vi "Self-Calibrate.vi"(8 "error in (no error)":errorcluster, 10 "Timeout (180000)":u32=180000, 11 "VISA resource name":refnum<visa-resource-name>) -> (0 "error out":errorcluster, 2 "Calibration Result":i32, 3 "VISA resource name out":refnum<visa-resource-name>)   [LabVIEW 2015, in "Tektronix TDS 200 1000 2000 Series.lvlib"]
doc: "Calibrates the oscilliscope for acquisitions and measurements."
uses:
  <instrlib>/Tektronix TDS 200 1000 2000 Series/Tektronix TDS 200 1000 2000 Series.lvlib
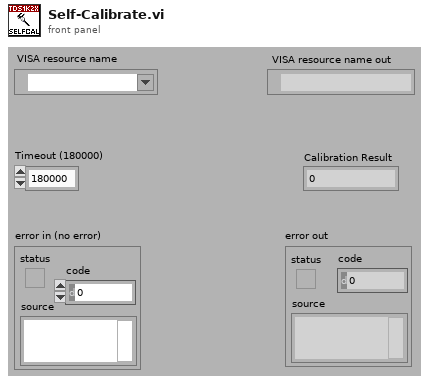
[diagram p1: front panel]
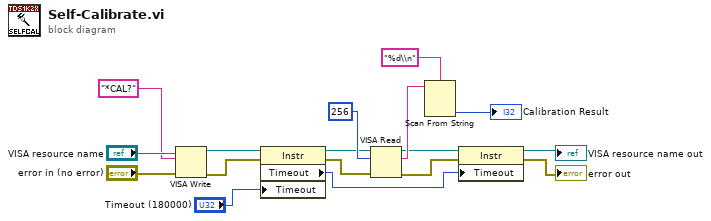
[diagram p0: block diagram]
diagram:
  n1 = VISA Write(VISA resource name="VISA resource name", write buffer="*CAL?", error in (no error)="error in (no error)") -> (VISA resource name out=w10:refnum<visa-resource-name>, error out=w7:errorcluster)  [unwired: 1 out]
  n2 = property class="Instr"(reference=w10, error in=w7, "Timeout"="Timeout (180000)") -> (reference out=w9:refnum<visa-resource-name>, error out=w8:errorcluster, "Timeout"=w2:u32)
  n3 = VISA Read(VISA resource name=w9, byte count=u32 256, error in (no error)=w8) -> (VISA resource name out=w6:refnum<visa-resource-name>, read buffer=w14:string, error out=w5:errorcluster)  [unwired: 1 out]
  n4 = Scan From String(format string="%d\\n", input string=w14) -> (output 1=→"Calibration Result":i32)  [unwired: 2 in, 4 out]
  n5 = property class="Instr"(reference=w6, error in=w5, "Timeout"=w2) -> (reference out=→"VISA resource name out":refnum<visa-resource-name>, error out=→"error out":errorcluster)
